vi "Axis_calibration_cluster.vi"() -> ()   [LabVIEW 2013]
doc: "This global variable stores the calibration data for the translation table axis motors, specifically the dead\nzone limits for each axis."
panel:
  in  "Dead-Zone Limits":T1={"Min neg. X"=-60.0, "Max neg. X"=-99.0, "Min pos. X"=63.0, "Max pos. X"=99.0, "Min neg. Y"=-30.0, "Max neg. Y"=-99.0, "Min pos. Y"=30.0, "Max pos. Y"=99.0, "Min neg. Z"=-13.0, "Max neg. Z"=-89.9, "Min pos. Z"=23.0, "Max pos. Z"=89.9, "Min neg. W"=-30.0, "Max neg. W"=-99.0, "Min pos. W"=30.0, "Max pos. W"=99.0}
  # "This global variable stores the calibration data for the translation table axis motors, specifically the dead\nzone limits for each axis."
  # "Note: max values are based on\ncounter settings and should not\nbe changed."
  # "Calibrated so far:\nMin neg. X\nMin pos. X\nMin neg. Z\nMin pos. Z"
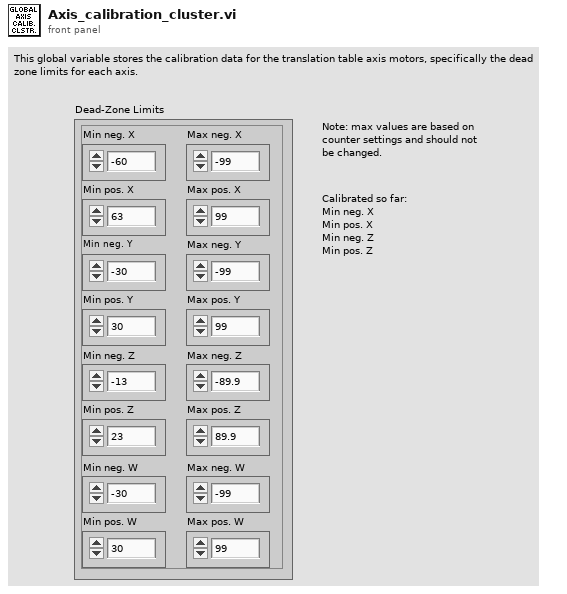
[diagram p1: front panel]
types:
  T1 = cluster{"Min neg. X":dbl, "Max neg. X":dbl, "Min pos. X":dbl, "Max pos. X":dbl, "Min neg. Y":dbl, "Max neg. Y":dbl, "Min pos. Y":dbl, "Max pos. Y":dbl, "Min neg. Z":dbl, "Max neg. Z":dbl, "Min pos. Z":dbl, "Max pos. Z":dbl, "Min neg. W":dbl, "Max neg. W":dbl, "Min pos. W":dbl, "Max pos. W":dbl}
diagram:
